vi "_ROSDefinition.vi"() -> ()   [LabVIEW 2010]
uses:
  <userlib>/ROSforLV_0.1/ROS/Code/SubVIs/_ROSDirection.ctl
panel:
  out "Ports":u16[](array[numeric])
  in  "FIFO Size":i32=10
  in  "Active Servers":T1(array[cluster])
  in  "Baxter Topics":T3(array[cluster])=[{"Topic"="/robot/head/command_head_nod", "Type"="std_msgs/Bool", "Action"=enum."Publisher"}, {"Topic"="/robot/limb/left/joint_command_mode", "Type"="baxter_msgs/JointCommandMode", "Action"=enum."Publisher"}, {"Topic"="/robot/limb/left/command_joint_angles", "Type"="baxter_msgs/JointPositions", "Action"=enum."Publisher"}, {"Topic"="/robot/limb/right/joint_command_mode", "Type"="baxter_msgs/JointCommandMode", "Action"=enum."Publisher"}, {"Topic"="/robot/limb/right/command_joint_angles", "Type"="baxter_msgs/JointPositions", "Action"=enum."Publisher"}, {"Topic"="/robot/set_super_enable", "Type"="std_msgs/Bool", "Action"=enum."Publisher"}, {"Topic"="/robot/joint_states", "Type"="sensor_msgs/JointState", "Action"=enum."Subscriber"}, {"Topic"="/robot/range/right_hand_range", "Type"="sensor_msgs/Range", "Action"=enum."Subscriber"}, {"Topic"="/robot/range/left_hand_range", "Type"="sensor_msgs/Range", "Action"=enum."Subscriber"}, {"Topic"="/cameras/left_hand_camera/image", "Type"="sensor_msgs/Image", "Action"=enum."Subscriber"}, {"Topic"="/cameras/right_hand_camera/image", "Type"="sensor_msgs/Image", "Action"=enum."Subscriber"}, {"Topic"="/cameras/head_camera/image", "Type"="sensor_msgs/Image", "Action"=enum."Subscriber"}, {"Topic"="/robot/limb/right/accessory/gripper/command_calibrate", "Type"="std_msgs/Bool", "Action"=enum."Publisher"}, {"Topic"="/robot/limb/left/accessory/gripper/command_calibrate", "Type"="std_msgs/Empty", "Action"=enum."Publisher"}, {"Topic"="/robot/limb/left/accessory/gripper/command_goto", "Type"="std_msgs/Float32", "Action"=enum."Publisher"}, {"Topic"="/robot/limb/right/accessory/gripper/command_goto", "Type"="std_msgs/Float32", "Action"=enum."Publisher"}, {"Topic"="/sdk/robot/digital_io/left_lower_cuff/state", "Type"="baxter_msgs/DigitalIOState", "Action"=enum."Subscriber"}, {"Topic"="/sdk/robot/digital_io/right_lower_cuff/state", "Type"="baxter_msgs/DigitalIOState", "Action"=enum."Subscriber"}, {"Topic"="/sdk/robot/digital_io/command", "Type"="baxter_msgs/DigitalOutputCommand", "Action"=enum."Publisher"}, {"Topic"="/sdk/robot/itb/torso_left_itb/state", "Type"="baxter_msgs/ITB", "Action"=enum."Subscriber"}, {"Topic"="/sdk/robot/itb/left_itb/state", "Type"="baxter_msgs/ITB", "Action"=enum."Subscriber"}, {"Topic"="/sdk/robot/itb/torso_right_itb/state", "Type"="baxter_msgs/ITB", "Action"=enum."Subscriber"}, {"Topic"="/sdk/robot/itb/right_itb/state", "Type"="baxter_msgs/ITB", "Action"=enum."Subscriber"}, {"Topic"="/sdk/xdisplay", "Type"="sensor_msgs/Image", "Action"=enum."Publisher"}, {"Topic"="/sdk/robot/digital_io/left_lower_button/state", "Type"="baxter_msgs/DigitalIOState", "Action"=enum."Subscriber"}, {"Topic"="/sdk/robot/digital_io/right_lower_button/state", "Type"="baxter_msgs/DigitalIOState", "Action"=enum."Subscriber"}, {"Topic"="/sdk/robot/digital_io/left_upper_button/state", "Type"="baxter_msgs/DigitalIOState", "Action"=enum."Subscriber"}, {"Topic"="/sdk/robot/digital_io/right_upper_button/state", "Type"="baxter_msgs/DigitalIOState", "Action"=enum."Subscriber"}, {"Topic"="/sdk/robot/limb/right/endpoint/state", "Type"="baxter_msgs/EndpointState", "Action"=enum."Subscriber"}, {"Topic"="/sdk/robot/limb/left/endpoint/state", "Type"="baxter_msgs/EndpointState", "Action"=enum."Subscriber"}, {"Topic"="/sdk/robot/limb/left/accessory/gripper/state", "Type"="baxter_msgs/GripperState", "Action"=enum."Subscriber"}, {"Topic"="/sdk/robot/limb/right/accessory/gripper/state", "Type"="baxter_msgs/GripperState", "Action"=enum."Subscriber"}, {"Topic"="/joint_states", "Type"="sensor_msgs/JointState", "Action"=enum."Subscriber"}, {"Topic"="/sdk/robot/limb/left/solve_ik_position", "Type"="baxter_msgs/SolvePositionIK", "Action"=enum."Service Client"}, {"Topic"="/sdk/robot/limb/right/solve_ik_position", "Type"="baxter_msgs/SolvePositionIK", "Action"=enum."Service Client"}, {"Topic"="/cameras/close", "Type"="baxter_msgs/CloseCamera", "Action"=enum."Service Client"}, {"Topic"="/cameras/open", "Type"="baxter_msgs/OpenCamera", "Action"=enum."Service Client"}, {"Topic"="/cameras/list", "Type"="baxter_msgs/ListCameras", "Action"=enum."Service Client"}, {"Topic"="/robot/sonar/head_sonar/state", "Type"="sensor_msgs/PointCloud", "Action"=enum."Subscriber"}, {"Topic"="/robot/limb/left/command_joint_velocities", "Type"="std_msgs/JointVelocities", "Action"=enum."Publisher"}, {"Topic"="/robot/limb/right/command_joint_velocities", "Type"="std_msgs/JointVelocities", "Action"=enum."Publisher"}, {"Topic"="/robot/sonar/set_lights", "Type"="std_msgs/uint16", "Action"=enum."Publisher"}, {"Topic"="/robot/sonar/set_red_level", "Type"="std_msgs/Float32", "Action"=enum."Publisher"}]
  in  "Nodes":cluster{"node":string, "Node Port":u32}[](array[cluster])=[{"node"="/labview", "Node Port"=7000}]
  out "Baxter There?":bool=TRUE
  out "ROS Master":string="192.168.1.110:11311"
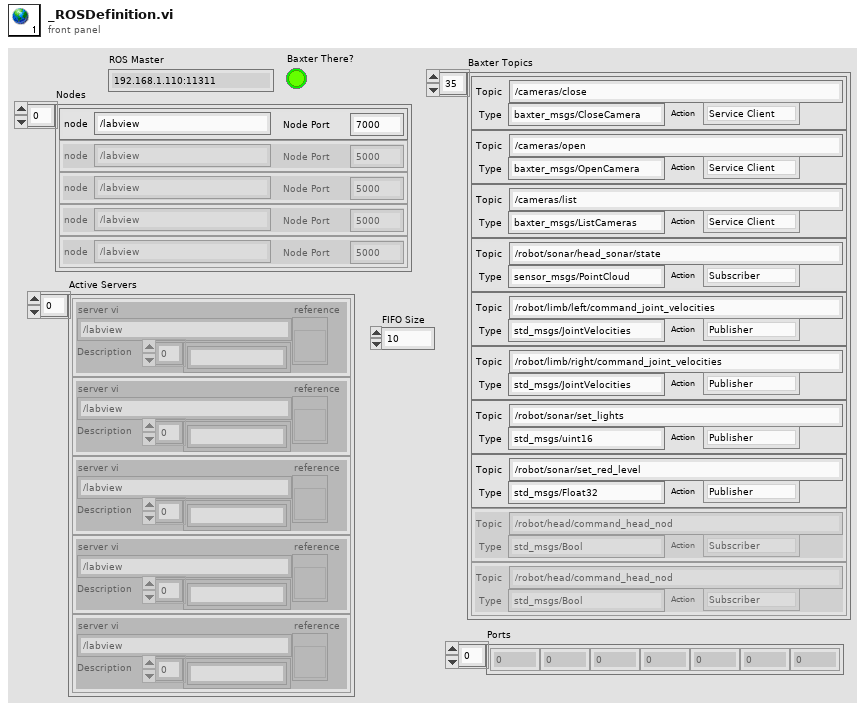
[diagram p1: front panel]
types:
  T1 = cluster{"server vi":string, "reference":refnum<vi>, "Description":string[]}[]
  T2 = typedef "_ROSDirection.ctl" = enum16{"Node", "Publisher", "Subscriber", "Service Client"}
  T3 = cluster{"Topic":string, "Type":string, "Action":T2}[]
diagram:
